vi "Initialize to Existing File.vi"() -> ()   [LabVIEW 2018]
uses:
  src/api/logger_class/Log Levels.ctl
  bc269cd9-d162-4013-a312-bd866d79ee19.vi
  src/api/configuration/handlers/file_handler/File Handler.lvclass
  C:/Users/Colin/Documents/software_projects/labview/glog/src/api/extension/formatting_handler_interface/Formatting Handler.lvclass
  src/api/logger_class/Log (Parts).vi
  src/api/logger_class/Logger.lvclass
panel:
  in  "initial filename":string
  in  "file name format":string="logfile_testing.log"
  out "error out":errorcluster
  in  "Stop":bool
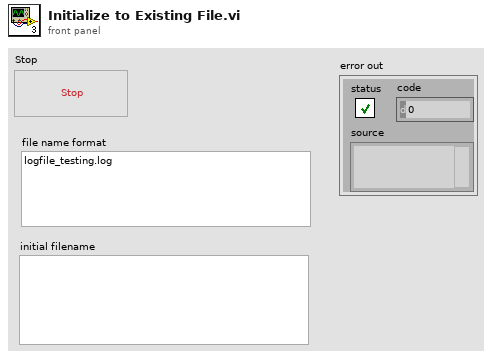
[diagram p1: front panel]
types:
  T1 = enum16{"open", "replace", "create", "open or create", "replace or create", "replace or create with confirmation"}
  T2 = typedef "GLog.lvlib/Logger.lvclass/Log Levels.ctl" = enum16{"Trace", "Debug", "Info", "Warning", "Error", "Critical"}
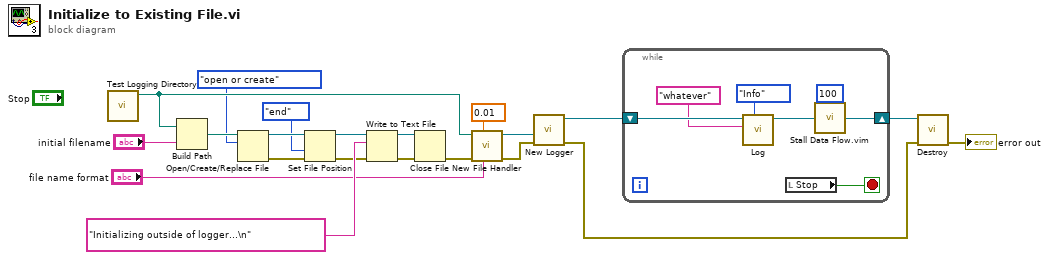
[diagram p0: block diagram]
diagram:
  n1 = call "Test Logging Directory.vi"() -> ("test logging directory"=w17:path)  [unwired: 11 in]
  n2 = Build Path(base path=w17, name or relative path="initial filename") -> (appended path=w18:path)
  n3 = Open/Create/Replace File(file path (use dialog)=w18, operation (0:open)=T1."open or create") -> (refnum out=w8:refnum<file>, error out=w6:errorcluster)  [unwired: 4 in, 1 out]
  n4 = Set File Position(refnum=w8, from (0:start)=enum16{"start", "end", "current"}."end", error in=w6) -> (refnum out=w9:refnum<file>, error out=w5:errorcluster)  [unwired: 1 in]
  n5 = Write to Text File(file (use dialog)=w9, text="Initializing outside of logger...\n", error in=w5) -> (refnum out=w14:refnum<file>, error out=w15:errorcluster)  [unwired: 1 in, 1 out]
  n6 = Close File(refnum=w14, error in=w15) -> (error out=w13:errorcluster)  [unwired: 1 out]
  n7 = call "New File Handler.vi"("file name format (\"logfile_%<%Y-%m-%d_%H-%M-%S>T.log\")"="file name format", "max file size [MB](50)"=0.01, "error in"=w13, "log directory (<app dir>/logs)"=w17) -> ("error out"=w12:errorcluster, "file handler"=w21:refnum<class "File Handler.lvclass">)  [unwired: 5 in, 1 out]
  n8 = call "New Logger.vi"("error in (no error)"=w12, "log handler (file handler)"=w21) -> ("error out"=w11:errorcluster, "logger"=w20:refnum<class "Logger.lvclass">)  [unwired: 8 in]
  n9 = while {
    shift-right: [w25] -> w19
    shift-left: w20 -> [w28]
    stop <- w23 stop-if-true
    n10 = call-poly "Log.vi"("log level"=Log_Levels."Info", "message"="whatever", "logger in"=w28) -> ("logger out"=w26:refnum<class "Logger.lvclass">)  [unwired: 8 in]
    n11 = local read "Stop"() -> (w23:bool)
    n12 = call "Stall Data Flow.vim"("value in"=w26, "milliseconds to wait"=u32 100) -> ("value out"=w25:refnum<class "Logger.lvclass">)  [unwired: 1 out]
  }
  n13 = call "Destroy.vi"("error in (no error)"=w11, "logger in"=w19) -> ("error out"=→"error out":errorcluster)  [unwired: 8 in, 1 out]
